vi "Log Result.vi"(8 "error in (no error)":errorcluster, 10 "tdms file":refnum<k34>, 11 "1D wfm (DBL) Result in":refnum<class "1D wfm (DBL) Result.lvclass">) -> (0 "error out":errorcluster, 2 "tdms file out":refnum<k34>, 3 "1D wfm (DBL) Result out":refnum<class "1D wfm (DBL) Result.lvclass">)   [LabVIEW 2015, in "1D wfm (DBL) Result.lvclass"]
uses:
  1D wfm (DBL) Result.lvclass
  Mag Lab Result.lvclass/Mag Lab Result.ctl
  1D wfm (DBL) Result.lvclass/1D wfm (DBL) Result.ctl
  Read Group Name.vi
  Read Name.vi
  Read Waveform data.vi
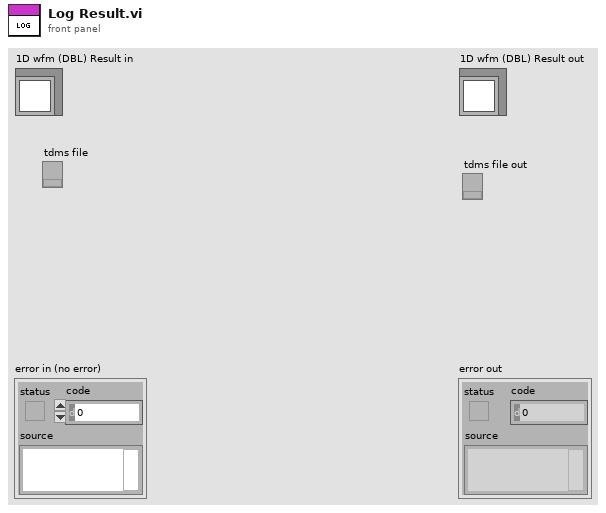
[diagram p1: front panel]
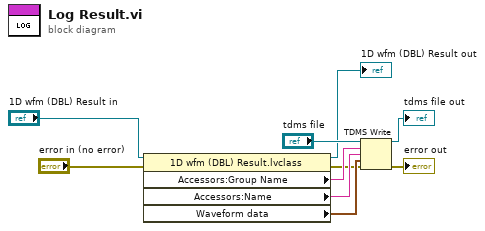
[diagram p0: block diagram]
diagram:
  n1 = property class="1D wfm (DBL) Result.lvclass"(reference="1D wfm (DBL) Result in", error in="error in (no error)") -> (reference out=→"1D wfm (DBL) Result out":refnum<class "1D wfm (DBL) Result.lvclass">, error out=w1:errorcluster, "Accessors:Group Name"=w4:string, "Accessors:Name"=w5:string, "Waveform data"=w6:waveform(dbl))
  n2 = TDMS Write(0:"tdms file", 5:w4, 7:w5, 9:w6, 11:w1) -> (4:→"tdms file out":refnum<k34>, 15:→"error out":errorcluster)  [unwired: 1 in, 2 out]
